vi "Get DIO configuration.vi"(8 "error in (no error)":errorcluster) -> (0 "error out":errorcluster, 2 "DO":T1, 3 "DI":T2)   [LabVIEW 2023]
uses:
  DI signals.ctl
  DO signals.ctl
  <vilib>/Utility/config.llb/Read Key (U32).vi
  <vilib>/Utility/config.llb/NI_LVConfig.lvlib
panel:
  out "error IO 2":errorcluster
  out "error IO":errorcluster
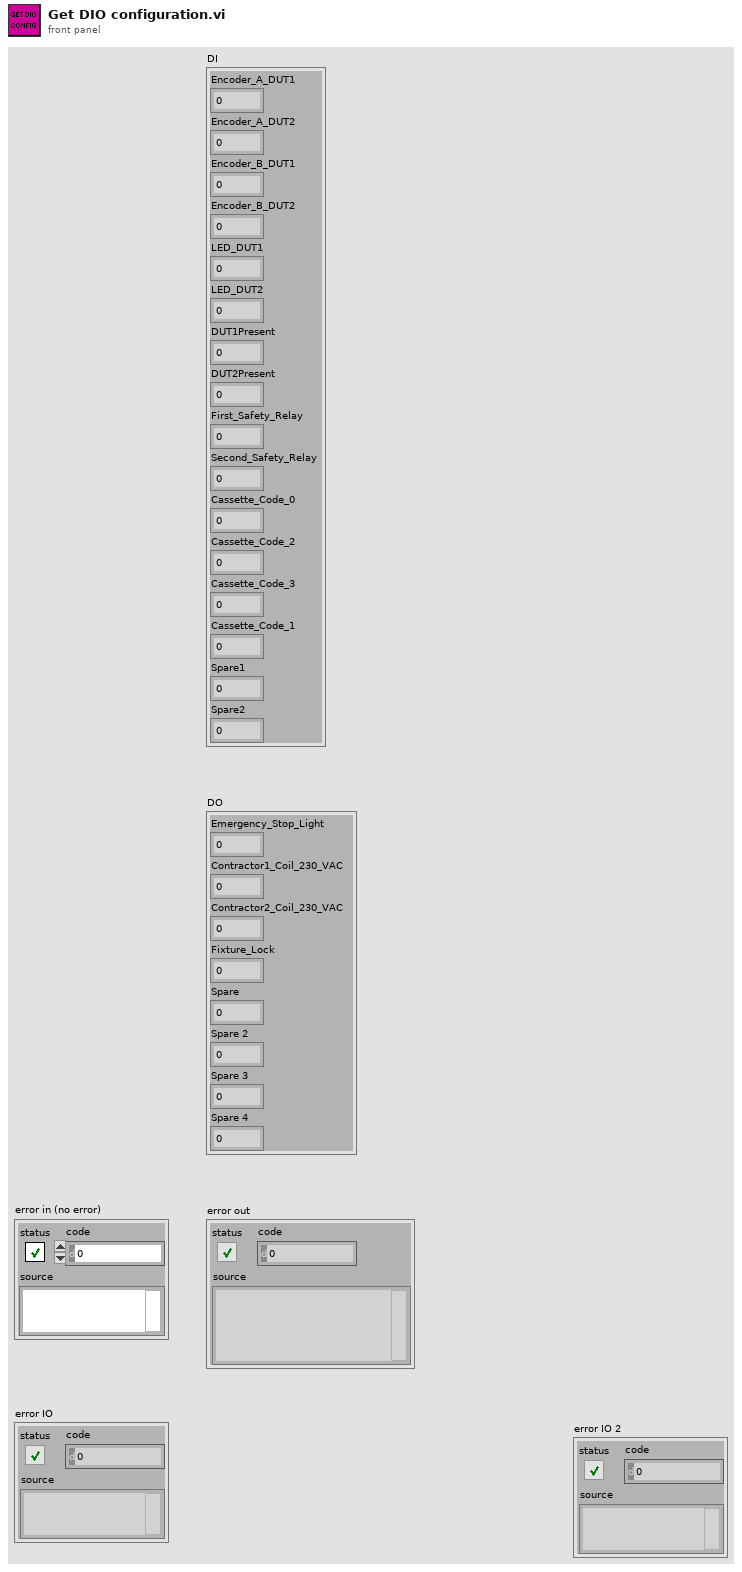
[diagram p1: front panel]
types:
  T1 = typedef "DO signals.ctl" = cluster{"Emergency_Stop_Light":i32, "Contractor1_Coil_230_VAC":i32, "Contractor2_Coil_230_VAC":i32, "Fixture_Lock":i32, "Spare":i32, "Spare 2":i32, "Spare 3":i32, "Spare 4":i32}
  T2 = typedef "DI signals.ctl" = cluster{"Encoder_A_DUT1":i32, "Encoder_A_DUT2":i32, "Encoder_B_DUT1":i32, "Encoder_B_DUT2":i32, "LED_DUT1":i32, "LED_DUT2":i32, "DUT1Present":i32, "DUT2Present":i32, "First_Safety_Relay":i32, "Second_Safety_Relay":i32, "Cassette_Code_0":i32, "Cassette_Code_2":i32, "Cassette_Code_3":i32, "Cassette_Code_1":i32, "Spare1":i32, "Spare2":i32}
  T3 = typedef "NI_LVConfig.lvlib/Config Data RefNum.ctl" = refnum<k1>
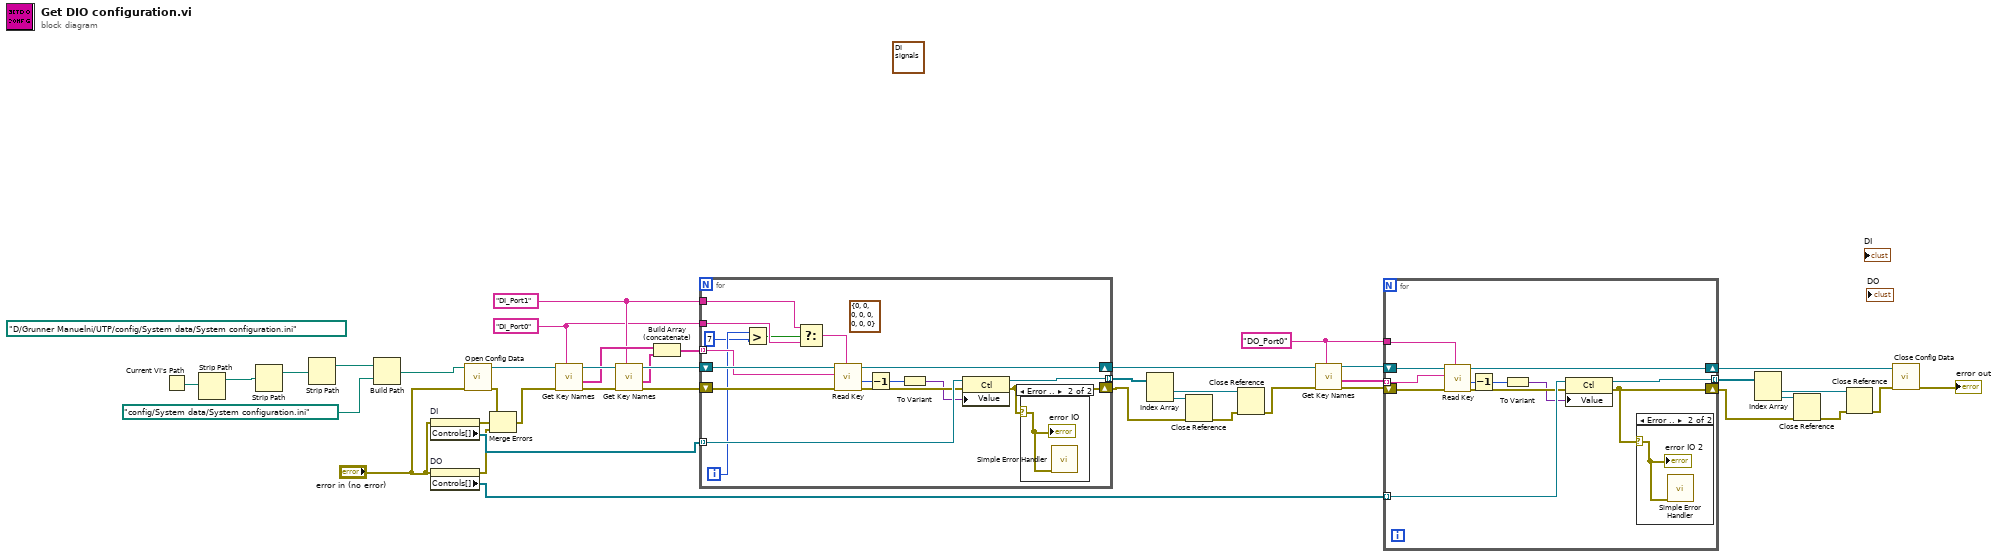
[diagram p0: block diagram]
diagram:
  w2 = "DI_Port1" ("section")
  w28 = "DO_Port0" ("section")
  w1 = "DI_Port0" ("section")
  (unwired) T2 {"Encoder_A_DUT1"=0, "Encoder_A_DUT2"=0, "Encoder_B_DUT1"=0, "Encoder_B_DUT2"=0, "LED_DUT1"=0, "LED_DUT2"=0, "DUT1Present"=0, "DUT2Present"=0, "First_Safety_Relay"=0, "Second_Safety_Relay"=0, "Cassette_Code_0"=0, "Cassette_Code_2"=0, "Cassette_Code_3"=0, "Cassette_Code_1"=0, "Spare1"=0, "Spare2"=0} ("DI")
  (unwired) path "D:/Grunner Manuelni/UTP/config/System data/System configuration.ini" ("configuration file path")
  n1 = Current VI's Path() -> (path=w12:path)
  n2 = Strip Path(path=w12) -> (stripped path=w11:path)  [unwired: 1 out]
  n3 = Strip Path(path=w11) -> (stripped path=w15:path)  [unwired: 1 out]
  n4 = Strip Path(path=w15) -> (stripped path=w14:path)  [unwired: 1 out]
  n5 = Build Path(base path=w14, name or relative path=path "config/System data/System configuration.ini") -> (appended path=w10:path)
  n6 = property on="DI" class="Clust (strict)"(error in="error in (no error)") -> (error out=w32:errorcluster, "Controls[]"=w33:refnum<vi>[])  [unwired: 1 in, 1 out]
  n7 = property on="DO" class="Clust (strict)"(error in="error in (no error)") -> (error out=w30:errorcluster, "Controls[]"=w29:refnum<vi>[])  [unwired: 1 in, 1 out]
  n8 = call <vilib>:"Open Config Data.vi"("error in (no error)"="error in (no error)", "configuration file path"=w10) -> ("error out"=w39:errorcluster, "refnum"=w42:T3)  [unwired: 7 in, 1 out]
  n9 = Merge Errors(w39, w32, w30) -> (w40:errorcluster)
  n10 = call <vilib>:"Get Key Names.vi"("section"=w1, "error in (no error)"=w40, "refnum"=w42) -> ("error out"=w9:errorcluster, "key names"=w5:string[], "refnum out"=w8:T3)  [unwired: 5 in, 1 out]
  n11 = call <vilib>:"Get Key Names.vi"("section"=w2, "error in (no error)"=w9, "refnum"=w8) -> ("error out"=w6:errorcluster, "key names"=w4:string[], "refnum out"=w7:T3)  [unwired: 5 in, 1 out]
  n12 = Build Array (concatenate)(w5, w4) -> (w3:string[])
  n13 = for {
    tunnel: w3 -> [w57] mode=indexing
    shift-right: [w58] -> w24
    shift-left: w7 -> [w59]
    tunnel: w33 -> [w55] mode=indexing
    tunnel: [w51] -> w38 mode=indexing
    shift-right: [w50] -> w34
    shift-left: w6 -> [w56]
    tunnel: w2 -> [w46]
    tunnel: w1 -> [w45]
    i -> [w48]
    (unwired) T1 {"Emergency_Stop_Light"=0, "Contractor1_Coil_230_VAC"=0, "Contractor2_Coil_230_VAC"=0, "Fixture_Lock"=0, "Spare"=0, "Spare 2"=0, "Spare 3"=0, "Spare 4"=0} ("DO")
    n14 = Greater?(x=w48, y=7) -> (0:w44:bool)
    n15 = Select(t=w46, s=w44, f=w45) -> (s? t:f=w43:string)
    n16 = call-poly <vilib>:"Read Key.vi"("section"=w43, "error in (no error)"=w56, "key"=w57, "refnum"=w59) -> ("error out"=w54:errorcluster, "value"=w53:u32, "refnum out"=w58:T3)  [unwired: 4 in, 1 out]
    n17 = Decrement(x=w53) -> (x-1=w49:u32)
    n18 = To Variant(anything=w49) -> (Variant=w52:variant)
    n19 = property class="Ctl"(reference=w55, error in=w54, "Value"=w52) -> (reference out=w51:refnum<vi>, error out=w50:errorcluster)
    n20 = case shown="Error .." w50 {
      selector: w50 -> [_ w60]
      frame No Error {
      }
      frame Error {
        n21 = call <vilib>:"Simple Error Handler.vi"("error in (no error)"=w60) -> ()  [unwired: 4 in, 5 out]
        "error IO" <- w60
      }
    }
  }
  n22 = Index Array(array=w38) -> (element #1=w37:refnum<vi>, element #2=w36:refnum<vi>)  [unwired: 2 in]
  n23 = Close Reference(reference=w36, error in (no error)=w34) -> (error out=w35:errorcluster)
  n24 = Close Reference(reference=w37, error in (no error)=w35) -> (error out=w26:errorcluster)
  n25 = call <vilib>:"Get Key Names.vi"("section"=w28, "error in (no error)"=w26, "refnum"=w24) -> ("error out"=w25:errorcluster, "key names"=w27:string[], "refnum out"=w23:T3)  [unwired: 5 in, 1 out]
  n26 = for {
    tunnel: w27 -> [w70] mode=indexing
    shift-right: [w71] -> w22
    shift-left: w23 -> [w72]
    tunnel: w28 -> [w69]
    tunnel: w29 -> [w67] mode=indexing
    tunnel: [w63] -> w18 mode=indexing
    shift-right: [w62] -> w17
    shift-left: w25 -> [w68]
    n27 = call-poly <vilib>:"Read Key.vi"("section"=w69, "error in (no error)"=w68, "key"=w70, "refnum"=w72) -> ("error out"=w66:errorcluster, "value"=w65:u32, "refnum out"=w71:T3)  [unwired: 4 in, 1 out]
    n28 = Decrement(x=w65) -> (x-1=w61:u32)
    n29 = To Variant(anything=w61) -> (Variant=w64:variant)
    n30 = property class="Ctl"(reference=w67, error in=w66, "Value"=w64) -> (reference out=w63:refnum<vi>, error out=w62:errorcluster)
    n31 = case shown="Error .." w62 {
      selector: w62 -> [_ w73]
      frame No Error {
      }
      frame Error {
        n32 = call <vilib>:"Simple Error Handler.vi"("error in (no error)"=w73) -> ()  [unwired: 4 in, 5 out]
        "error IO 2" <- w73
      }
    }
  }
  n33 = Index Array(array=w18) -> (element #1=w19:refnum<vi>, element #2=w20:refnum<vi>)  [unwired: 2 in]
  n34 = Close Reference(reference=w20, error in (no error)=w17) -> (error out=w21:errorcluster)
  n35 = Close Reference(reference=w19, error in (no error)=w21) -> (error out=w16:errorcluster)
  n36 = call <vilib>:"Close Config Data.vi"("error in (no error)"=w16, "refnum"=w22) -> ("error out"=→"error out":errorcluster)  [unwired: 8 in, 1 out]
